vi "SET_POSITION_TARGET_LOCAL_NED.vi"(7 "MAV ID":u8, 9 "vz":sgl, 10 "vy":sgl, 11 "vx":sgl) -> (3 "MAVLink Message":u8[](array[numeric]))   [LabVIEW 2014]
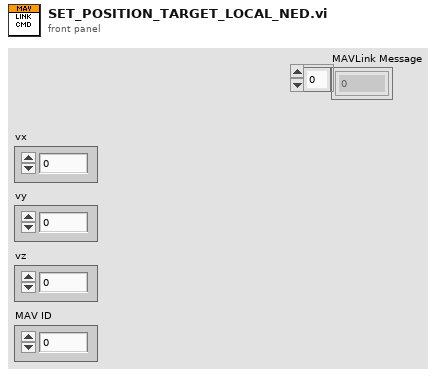
[diagram p1: front panel]
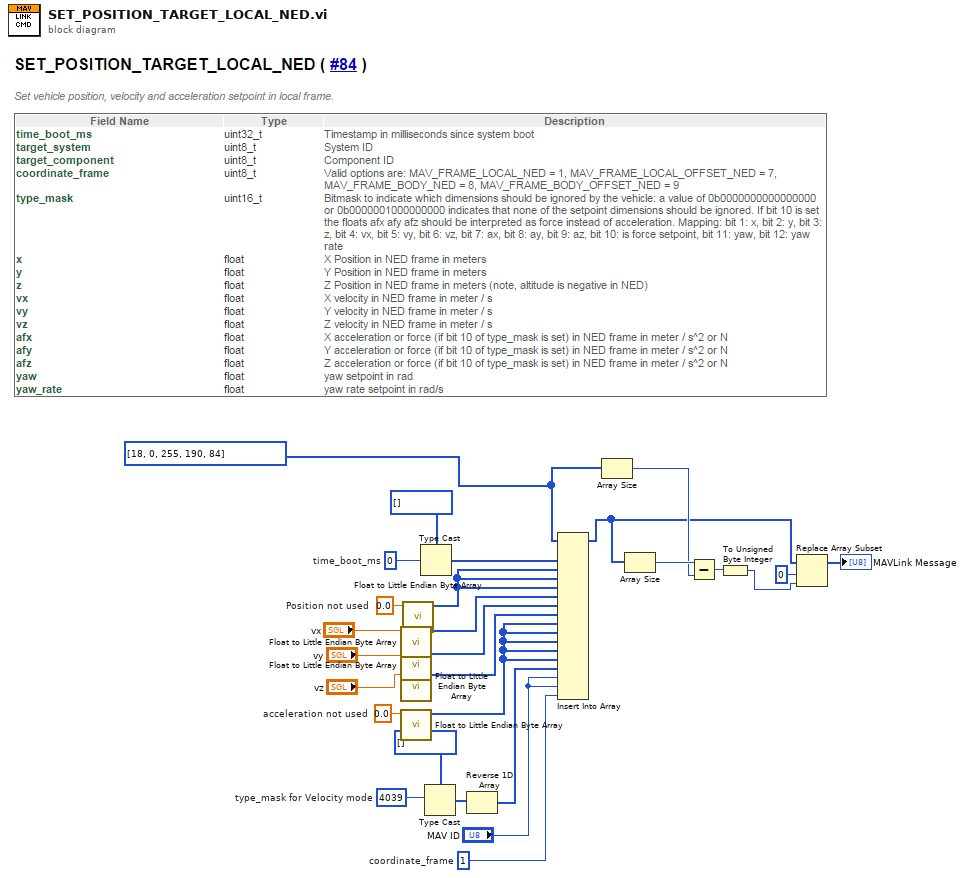
[diagram p0: block diagram]
diagram:
  w1 = u8 1  # coordinate_frame
  w5 = u16 4039  # type_mask for Velocity mode
  w8 = sgl 0.0  # acceleration not used
  w15 = sgl 0.0  # Position not used
  w18 = u32 0  # time_boot_ms
  w27 = u8[] [18, 0, 255, 190, 84]
  n1 = call "Float to Little Endian Byte Array.vi"("Float In"="vx") -> ("LE Byte Array"=w13:u8[])  [unwired: 10 in]
  n2 = call "Float to Little Endian Byte Array.vi"("Float In"="vy") -> ("LE Byte Array"=w11:u8[])  [unwired: 10 in]
  n3 = call "Float to Little Endian Byte Array.vi"("Float In"="vz") -> ("LE Byte Array"=w9:u8[])  [unwired: 10 in]
  n4 = call "Float to Little Endian Byte Array.vi"("Float In"=w8) -> ("LE Byte Array"=w7:u8[])  [unwired: 10 in]
  n5 = call "Float to Little Endian Byte Array.vi"("Float In"=w15) -> ("LE Byte Array"=w14:u8[])  [unwired: 10 in]
  n6 = Type Cast(type=u8[] [], x=w18) -> (*(type *) &x=w17:u8[])
  n7 = Type Cast(type=u8[] [], x=w5) -> (*(type *) &x=w4:u8[])
  n8 = Reverse 1D Array(array=w4) -> (reversed array=w3:u8[])
  n9 = Insert Into Array(array=w27, new element #1=w17, new element #2=w14, new element #3=w14, new element #4=w14, new element #5=w13, new element #6=w11, new element #7=w9, new element #8=w7, new element #9=w7, new element #10=w7, new element #11=w7, new element #12=w7, new element #13=w3, new element #14="MAV ID", new element #15="MAV ID", new element #16=w1) -> (w21:u8[])  [unwired: 1 in]
  n10 = Array Size(array=w27) -> (size(s)=w25:i32)
  n11 = Array Size(array=w21) -> (size(s)=w26:i32)
  n12 = Subtract(x=w26, y=w25) -> (x-y=w24:i32)
  n13 = To Unsigned Byte Integer(number=w24) -> (unsigned 8bit integer=w22:u8)
  n14 = Replace Array Subset(array=w21, new element=w22, index=0) -> (→"MAVLink Message":u8[])
